vi "Volume entry-Disable Z step ctrl.vi"(8 "error in (no error)":errorcluster) -> (0 "error out":errorcluster)   [LabVIEW 2020]
uses:
  ROI Entry screen/Globals/gl_Volume Entry UI globals.vi
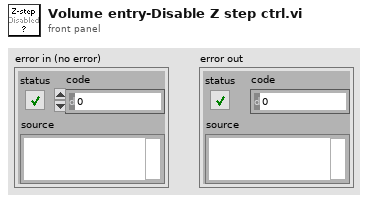
[diagram p1: front panel]
types:
  T1 = enum8{"Enabled", "Disabled", "Disabled and Grayed Out"}
  T2 = typedef "Volume entry ctrl refs cluster.ctl" = cluster{"Z-step (planes)":refnum<vi>, "Volume":refnum<vi>, "Dual Rectangle":refnum<vi>, "Zoom":refnum<vi>, "Z-plane 1":refnum<vi>, "Z-plane 2":refnum<vi>, "ZplaneIndex (zero based)":refnum<vi>}
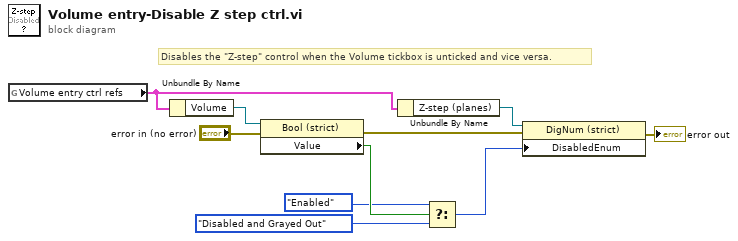
[diagram p0: block diagram]
diagram:
  # "Disables the \"Z-step\" control when the Volume tickbox is unticked and vice versa."
  n1 = global read "gl_Volume Entry UI globals.vi" "Volume entry ctrl refs"() -> (w6:T2)
  n2 = Unbundle By Name(w6) -> ("Volume"=w7:refnum<vi>)
  n3 = property on="Property Node" class="Bool (strict)"(reference=w7, error in="error in (no error)") -> (error out=w8:errorcluster, "Value"=w4:bool)  [unwired: 1 out]
  n4 = Unbundle By Name(w6) -> ("Z-step (planes)"=w5:refnum<vi>)
  n5 = Select(t=T1."Enabled" ("Disabled"), s=w4, f=T1."Disabled and Grayed Out" ("Disabled")) -> (s? t:f=w1:T1)
  n6 = property on="Property Node" class="DigNum (strict)"(reference=w5, error in=w8, "DisabledEnum"=w1) -> (error out=→"error out":errorcluster)  [unwired: 1 out]
